vi "LinkToBack.vi"(8 "error in (no error)":errorcluster, 10 "newBackNode":refnum<data-value>, 11 "LinkedList in":refnum<class "LinkedList.lvclass">) -> (0 "error out":errorcluster, 1 "ignored":bool, 3 "LinkedList out":refnum<class "LinkedList.lvclass">)   [LabVIEW 2014, in "LinkedList.lvlib" / "LinkedList.lvclass"]
doc: "Links a node to the back of the linked list."
uses:
  <userlib>/AdvancedDataStructures/ClassBased/LinkedList/LinkedList.lvclass
  <userlib>/AdvancedDataStructures/ClassBased/LLNode/LLNode.lvclass
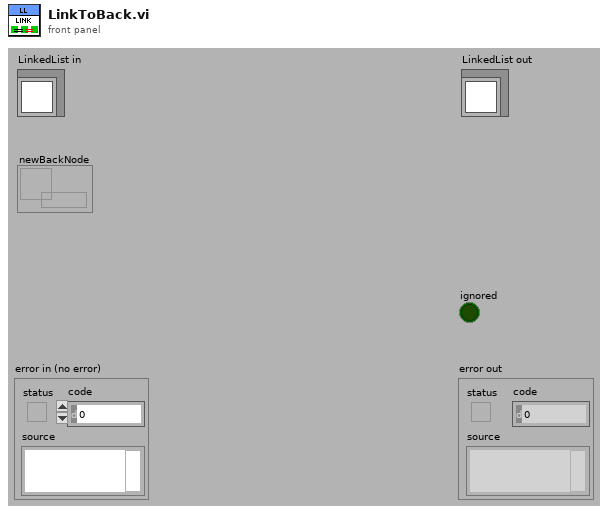
[diagram p1: front panel]
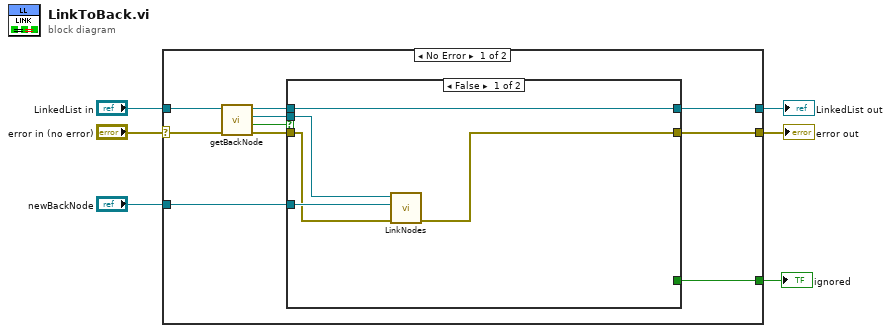
[diagram p0: block diagram]
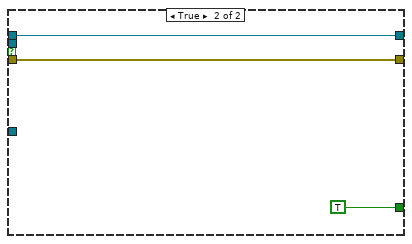
[diagram p2: hidden frame]
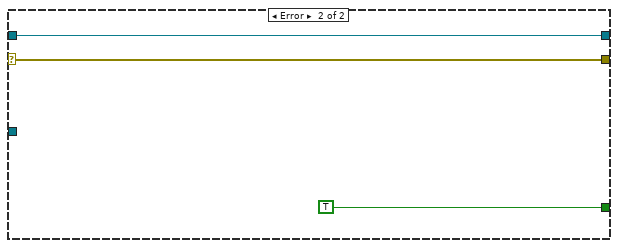
[diagram p3: hidden frame]
diagram:
  n1 = case shown="No Error" "error in (no error)" {
    selector: "error in (no error)" -> [w15 w26]
    tunnel: [w9 w27] -> w4
    tunnel: "LinkedList in" -> [w16 w27]
    tunnel: "newBackNode" -> [w8 _]
    tunnel: [w10 TRUE] -> w2
    tunnel: [w7 w26] -> w1
    frame No Error {
      n2 = call <userlib>:"getBackNode.vi"("error in (no error)"=w15, "LinkedList in"=w16) -> ("error out"=w11:errorcluster, "ignore"=w13:bool, "BackNode"=w12:refnum<data-value>, "LinkedList out"=w14:refnum<class "LinkedList.lvclass">)  [unwired: 6 in]
      n3 = case shown="False" w13 {
        tunnel: w14 -> [w21 w22]
        tunnel: w12 -> [w18 _]
        tunnel: w11 -> [w19 w23]
        tunnel: [_ TRUE] -> w10
        tunnel: [w21 w22] -> w9
        tunnel: w8 -> [w20 _]
        tunnel: [w17 w23] -> w7
        frame False {
          n4 = call <userlib>:"LinkNodes.vi"("error in (no error)"=w19, "NextNode in"=w20, "PreviousNode in"=w18) -> ("error out"=w17:errorcluster)  [unwired: 6 in, 2 out]
        }
        frame True {
        }
      }
    }
    frame Error {
    }
  }
  "error out" <- w1
  "LinkedList out" <- w4
  "ignored" <- w2
